vi "MAIN TRIAL CODE.vi"() -> ()   [LabVIEW 2025]
doc: "Use this template to build a producer/consumer design pattern with events to produce queue items. Use this design pattern instead of the User Interface Event Handler pattern for user interfaces when you want to execute code asynchronously in response to an event without slowing the user interface responsiveness."
panel:
  in  "timeout ms (25000)":i32=200
  out "Downlink Packet":T1
  out "buffer_overrun count":u32
  out "AE Ring-Down Counts":u32(graph)
  out "Last Config Rejected":u32
  out "rx command count":u32
  out "Current Filter Id":u32
  out "AE Ring-Down Counts":u32
  out "System Status":u32
  out "Timestamp":u32
  out "Sequence ID":u32
  out "Signal Energy":sgl(graph)
  out "Amplitude db_AE":sgl(graph)
  out "Peak Amplitude":sgl(graph)
  in  "Uplink Packet":T2
  in  "Send Command":bool
  out "Isolated Gain":u32
  out "DAQ Status":u32
  in  "Connect Sensor":bool
  in  "stop":bool
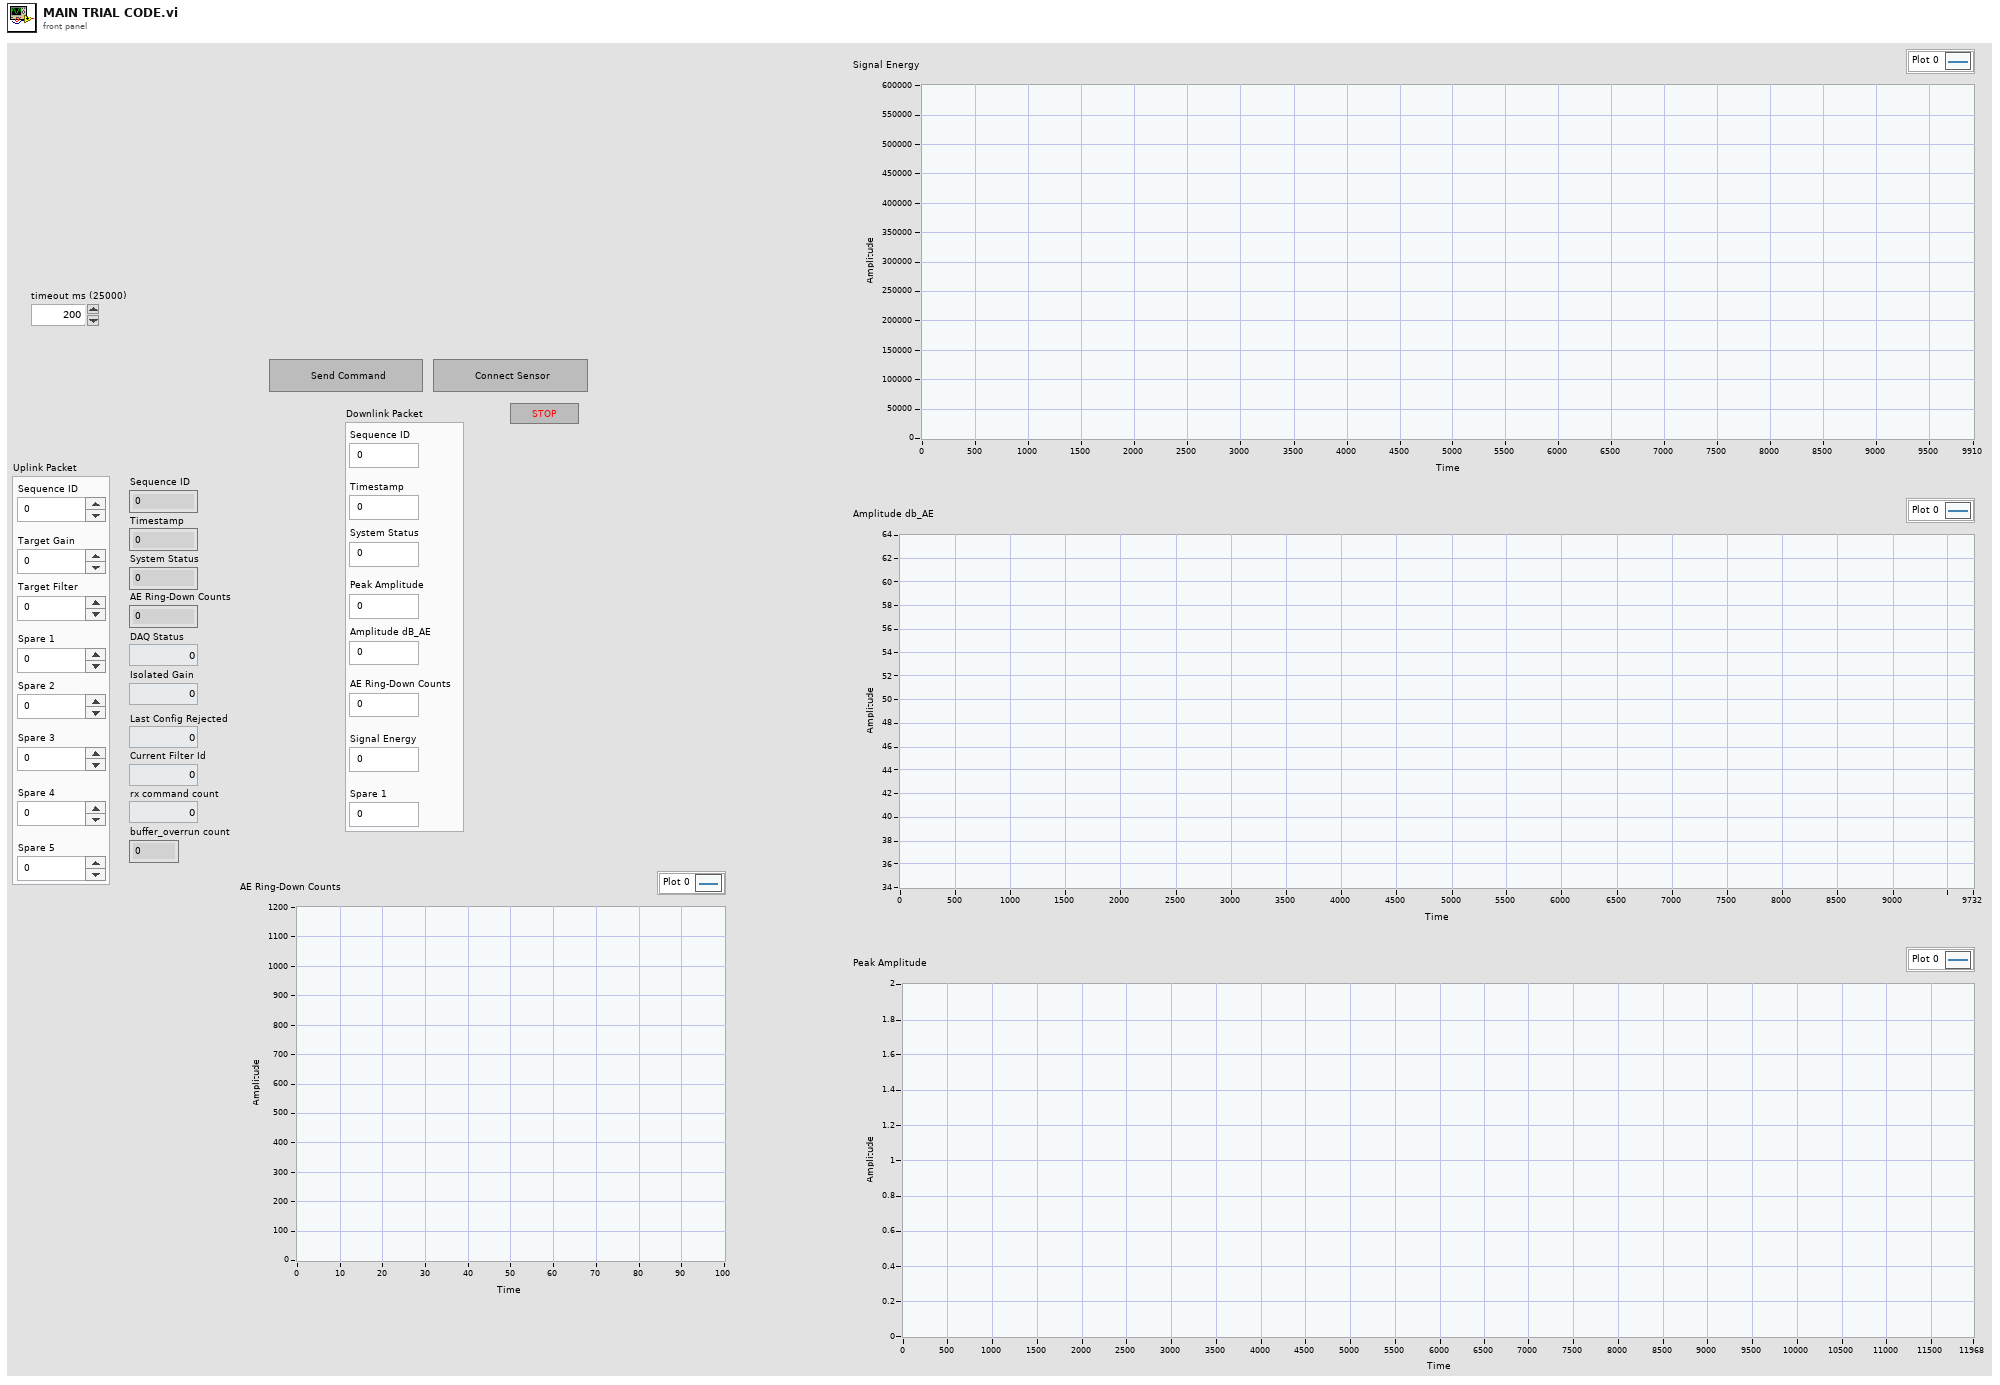
[diagram p1: front panel]
types:
  T1 = cluster{"Sequence ID":u32, "Timestamp":u32, "System Status":u32, "Peak Amplitude":u32, "Amplitude dB_AE":u32, "AE Ring-Down Counts":u32, "Signal Energy":u32, "Spare 1":u32}
  T2 = cluster{"Sequence ID":u32, "Target Gain":u32, "Target Filter":u32, "Spare 1":u32, "Spare 2":u32, "Spare 3":u32, "Spare 4":u32, "Spare 5":u32}
  T3 = cluster{"Sequence ID":u32, "Timestamp":u32, "System Status":u32, "Peak Amplitude":sgl, "Amplitude dB_AE":sgl, "AE Ring-Down Counts":u32, "Signal Energy":sgl, "Spare 1":u32}
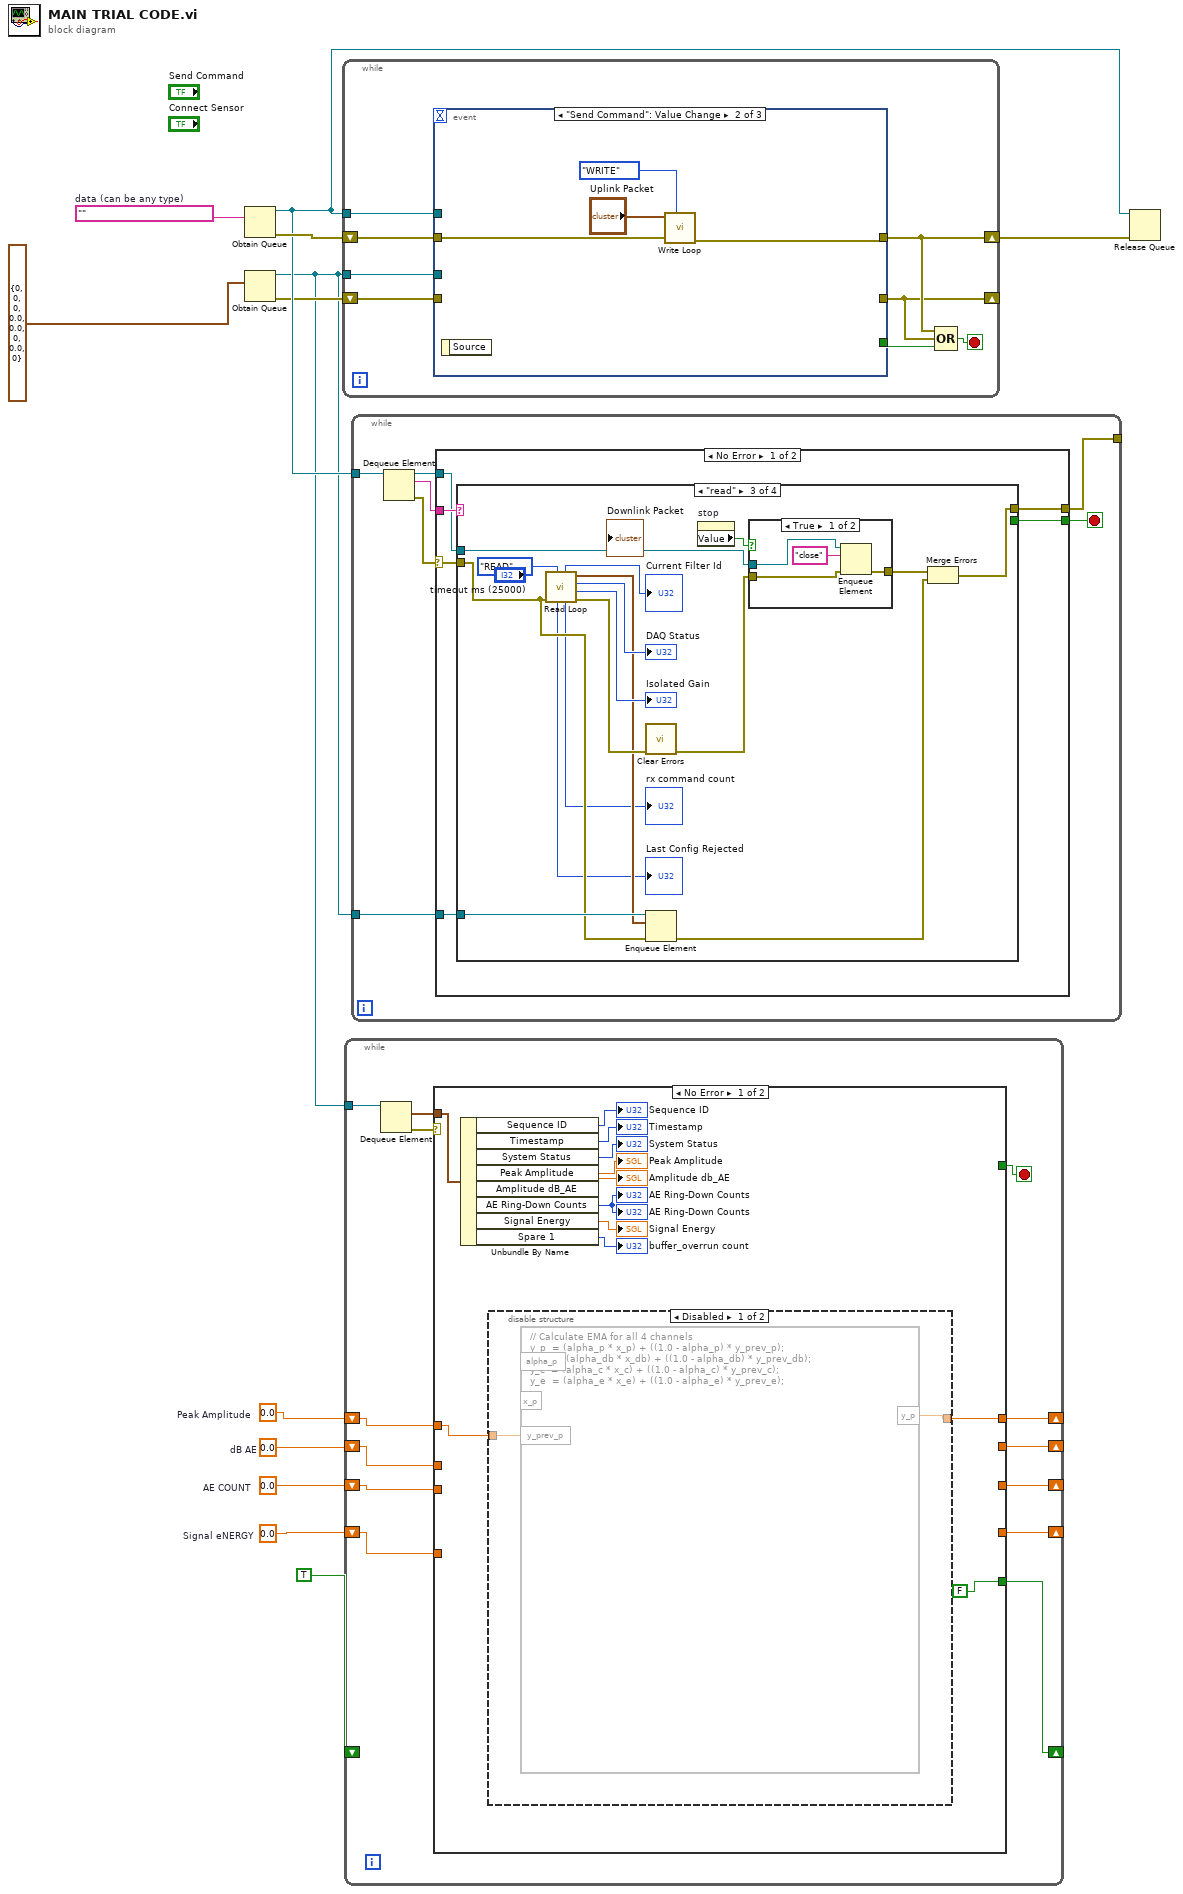
[diagram p0: block diagram]
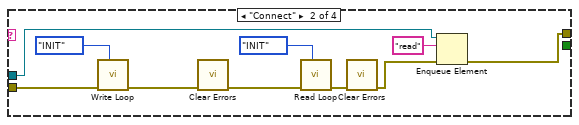
[diagram p3: hidden frame]
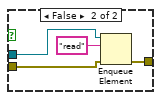
[diagram p4: hidden frame]
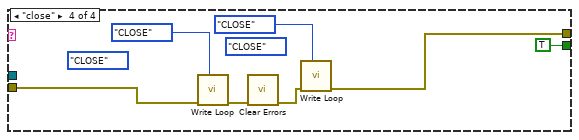
[diagram p5: hidden frame]
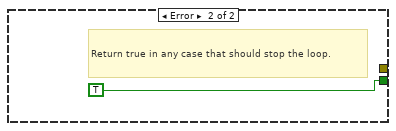
[diagram p6: hidden frame]
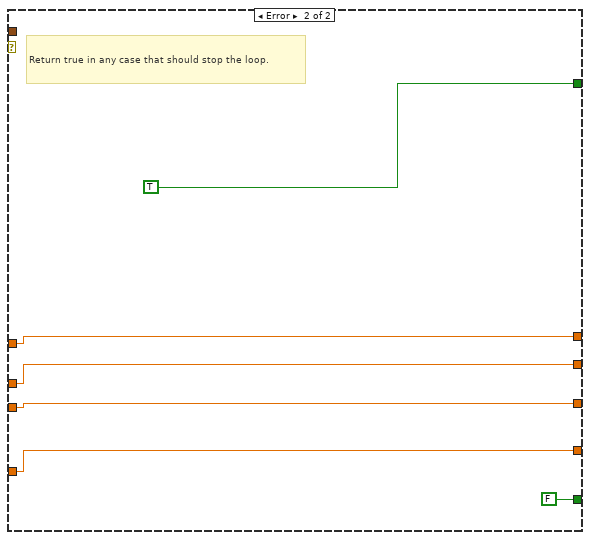
[diagram p8: hidden frame]
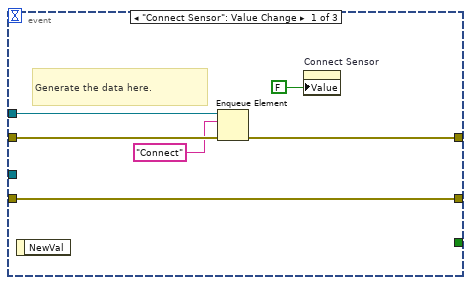
[diagram p9: hidden frame]
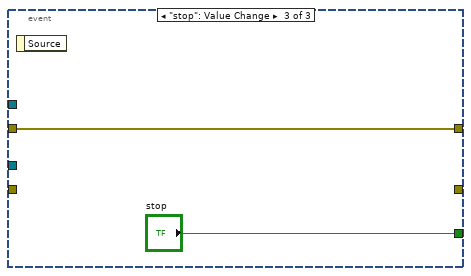
[diagram p10: hidden frame]
diagram:
  w1 = sgl 0.0  # Signal eNERGY
  w2 = sgl 0.0  # AE COUNT
  w3 = sgl 0.0  # dB AE
  w4 = sgl 0.0  # Peak Amplitude
  w10 = ""  # data (can be any type)
  n1 = Obtain Queue(element data type=w10) -> (queue out=w9:refnum<queue>, error out=w12:errorcluster)  [unwired: 4 in, 1 out]
  n2 = Obtain Queue(element data type=T3 {"Sequence ID"=0, "Timestamp"=0, "System Status"=0, "Peak Amplitude"=0.0, "Amplitude dB_AE"=0.0, "AE Ring-Down Counts"=0, "Signal Energy"=0.0, "Spare 1"=0} ("Downlink Packet")) -> (queue out=w7:refnum<queue>, error out=w8:errorcluster)  [unwired: 4 in, 1 out]
  n3 = while {
    shift-right: [w14] -> w11
    shift-left: w12 -> [w19]
    tunnel: w9 -> [w20]
    tunnel: w7 -> [w16]
    shift-right: [w13] -> _
    shift-left: w8 -> [w15]
    stop <- w17 stop-if-true
    n4 = event shown="[1] \"Send Command\": Value Change" {
      selector: _ -> [_ _ _]
      dyn-events: _ -> [_ _ _]
      timeout: _ -> [_ _ _]
      tunnel: w20 -> [w26 _ _]
      tunnel: w19 -> [w25 w30 w31]
      tunnel: [w24 w28 w31] -> w14
      tunnel: [_ _ "stop"] -> w18
      tunnel: w16 -> [_ _ _]
      tunnel: w15 -> [w22 _ _]
      tunnel: [w22 _ _] -> w13
      event "Connect Sensor": Value Change {
        # "Generate the data here."
        n5 = event-data() -> ()  [unwired: 1 in, 1 out]
        n6 = Enqueue Element(queue=w26, element="Connect", error in (no error)=w25) -> (error out=w24:errorcluster)  [unwired: 1 in, 2 out]
        n7 = property on="Connect Sensor" class="Bool (strict)"("Value"=FALSE ("Connect Sensor")) -> ()  [unwired: 2 in, 2 out]
      }
      event "Send Command": Value Change {
        n8 = event-data() -> ()  [unwired: 1 in, 1 out]
        n9 = call "Write Loop.vi"("Enum - Menu"=enum16{"INIT", "WRITE", "RE-INIT", "CLOSE"}."WRITE", "error in (no error)"=w30, "Uplink Packet"="Uplink Packet") -> ("error out"=w28:errorcluster)  [unwired: 8 in]
      }
      event "stop": Value Change {
        n10 = event-data() -> ()  [unwired: 1 in, 1 out]
      }
    }
    n11 = Compound Arithmetic op=OR(w14, w13, w18) -> (w17:bool)
  }
  n12 = while {
    tunnel: w7 -> [w45]
    shift-right: [w41] -> _
    shift-left: w4 -> [w40]
    shift-right: [w39] -> _
    shift-left: w3 -> [w38]
    shift-right: [w37] -> _
    shift-left: w2 -> [w36]
    shift-right: [w35] -> _
    shift-left: w1 -> [w34]
    shift-right: [w33] -> _
    shift-left: TRUE -> [_]
    stop <- w42 stop-if-true
    n13 = Dequeue Element(queue=w45) -> (element=w43:T3, error out=w44:errorcluster)  [unwired: 2 in, 2 out]
    n14 = case shown="No Error" w44 {
      tunnel: w43 -> [w57 _]
      tunnel: [_ TRUE] -> w42
      tunnel: [w46 w65] -> w41
      tunnel: w40 -> [w47 w65]
      tunnel: [_ w64] -> w39
      tunnel: w38 -> [_ w64]
      tunnel: [_ w63] -> w37
      tunnel: w36 -> [_ w63]
      tunnel: [_ w62] -> w35
      tunnel: w34 -> [_ w62]
      tunnel: [FALSE FALSE] -> w33
      frame No Error {
        n15 = Unbundle By Name(w57) -> ("Sequence ID"=→"Sequence ID":u32, "Timestamp"=→"Timestamp":u32, "System Status"=→"System Status":u32, "Peak Amplitude"=→"Peak Amplitude":sgl, "Amplitude dB_AE"=→"Amplitude db_AE":sgl, "AE Ring-Down Counts"=→"AE Ring-Down Counts" →"AE Ring-Down Counts":u32, "Signal Energy"=→"Signal Energy":sgl, "Spare 1"=→"buffer_overrun count":u32)
        n16 = disable-structure shown="Disabled" {
          disable-tunnel: w47 -> [w59 w60]
          disable-tunnel: [w58 w60] -> w46
          frame Disabled {
            n17 = formula code="// Calculate EMA for all 4 channels\ny_p  = (alpha_p * x_p) + ((1.0 - alpha_p) * y_prev_p);\ny_db = (alpha_db * x_db) + ((1.0 - alpha_db) * y_prev_db);\ny_c  = (alpha_c * x_c) + ((1.0 - alpha_c) * y_prev_c);\ny_e  = (alpha_e * x_e) + ((1.0 - alpha_e) * y_prev_e);"("y_prev_p"=w59) -> ("y_p"=w58:dbl)  [unwired: 2 in]
          }
          frame Enabled {
          }
        }
      }
      frame Error {
        # "Return true in any case that should stop the loop."
      }
    }
  }
  n18 = while {
    tunnel: w9 -> [w73]
    tunnel: [w68] -> _
    tunnel: w7 -> [w67]
    stop <- w70 stop-if-true
    n19 = Dequeue Element(queue=w73) -> (queue out=w69:refnum<queue>, element=w71:string, error out=w72:errorcluster)  [unwired: 2 in, 1 out]
    n20 = case shown="No Error" w72 {
      selector: w72 -> [w77 _]
      tunnel: w71 -> [w79 _]
      tunnel: [w75 TRUE] -> w70
      tunnel: w69 -> [w78 _]
      tunnel: [w76 _] -> w68
      tunnel: w67 -> [w74 _]
      frame No Error {
        n21 = case shown="\"read\"" w79 {
          tunnel: w78 -> [_ w89 w105 _]
          tunnel: w77 -> [w80 w88 w97 w121]
          tunnel: [w80 w85 w96 w118] -> w76
          tunnel: [_ _ _ TRUE] -> w75
          tunnel: w74 -> [_ _ w99 _]
          frame "False", Default {
          }
          frame "Connect" {
            n22 = call "Write Loop.vi"("Enum - Menu"=enum16{"INIT", "WRITE", "RE-INIT", "CLOSE"}."INIT", "error in (no error)"=w88) -> ("error out"=w87:errorcluster)  [unwired: 9 in]
            n23 = call <vilib>:"Clear Errors.vi"("error in (no error)"=w87) -> ("error out"=w84:errorcluster)  [unwired: 5 in, 1 out]
            n24 = call "Read Loop.vi"("Enum - Menu"=enum16{"INIT", "READ", "RE-INIT", "CLOSE"}."INIT", "error in (no error)"=w84) -> ("error out"=w83:errorcluster)  [unwired: 3 in, 6 out]
            n25 = call <vilib>:"Clear Errors.vi"("error in (no error)"=w83) -> ("error out"=w81:errorcluster)  [unwired: 5 in, 1 out]
            n26 = Enqueue Element(queue=w89, element="read", error in (no error)=w81) -> (error out=w85:errorcluster)  [unwired: 1 in, 2 out]
          }
          frame "read" {
            n27 = call "Read Loop.vi"("Enum - Menu"=enum16{"INIT", "READ", "RE-INIT", "CLOSE"}."READ", "error in (no error)"=w97) -> ("error out"=w104:errorcluster, "Isolated Gain"=→"Isolated Gain":u32, "DAQ Status"=→"DAQ Status":u32, "Downlink Packet"=w98:T1, "rx command count"=→"rx command count":u32, "Current Filter Id"=→"Current Filter Id":u32, "Last Config Rejected"=→"Last Config Rejected":u32)  [unwired: 3 in]
            n28 = call <vilib>:"Clear Errors.vi"("error in (no error)"=w104) -> ("error out"=w94:errorcluster)  [unwired: 5 in, 1 out]
            n29 = Enqueue Element(queue=w99, element=w98, error in (no error)=w97) -> (error out=w95:errorcluster)  [unwired: 1 in, 2 out]
            n30 = property on="stop" class="Bool (strict)"() -> ("Value"=w102:bool)  [unwired: 2 in, 2 out]
            n31 = case shown="True" w102 {
              tunnel: [w109 w113] -> w106
              tunnel: w105 -> [w108 w112]
              tunnel: w94 -> [w107 w111]
              frame True {
                n32 = Enqueue Element(queue=w108, element="close", error in (no error)=w107) -> (error out=w109:errorcluster)  [unwired: 1 in, 2 out]
              }
              frame False {
                n33 = Enqueue Element(queue=w112, element="read", error in (no error)=w111) -> (error out=w113:errorcluster)  [unwired: 1 in, 2 out]
              }
            }
            n34 = Merge Errors(w106, w95) -> (w96:errorcluster)
          }
          frame "close" {
            (unwired) enum16{"INIIT", "WRITE", "REINT", "CLOSE"}."CLOSE" ("Enum - Menu")
            (unwired) enum16{"INIIT", "WRITE", "REINT", "CLOSE"}."CLOSE" ("Enum - Menu")
            n35 = call "Write Loop.vi"("Enum - Menu"=enum16{"INIT", "WRITE", "RE-INIT", "CLOSE"}."CLOSE", "error in (no error)"=w121) -> ("error out"=w119:errorcluster)  [unwired: 9 in]
            n36 = call <vilib>:"Clear Errors.vi"("error in (no error)"=w119) -> ("error out"=w117:errorcluster)  [unwired: 5 in, 1 out]
            n37 = call "Write Loop.vi"("Enum - Menu"=enum16{"INIT", "WRITE", "RE-INIT", "CLOSE"}."CLOSE", "error in (no error)"=w117) -> ("error out"=w118:errorcluster)  [unwired: 9 in]
          }
        }
      }
      frame Error {
        # "Return true in any case that should stop the loop."
      }
    }
  }
  n38 = Release Queue(queue=w9, error in (no error)=w11) -> ()  [unwired: 1 in, 3 out]
